vi "Draw Scale.vi"(6 "scale color":u32(colorbox), 9 "draw area cache":T1, 10 "heading (deg)":dbl, 11 "picture in":picture) -> (3 "picture out":picture)   [LabVIEW 2017, in "NI_Robotics_Compass Picture.lvlib"]
uses:
  <vilib>/robotics/Controls/Compass Indicator/Compass Picture/NI_Robotics_Compass Picture.lvlib
  <vilib>/robotics/Controls/Compass Indicator/Compass Picture/Draw Area State.ctl
  <vilib>/Utility/miscctls.llb/LVBoundsTypeDef.ctl
  <vilib>/picture/picture.llb/Draw Text at Point.vi
  <vilib>/picture/picture.llb/Draw Multiple Lines.vi
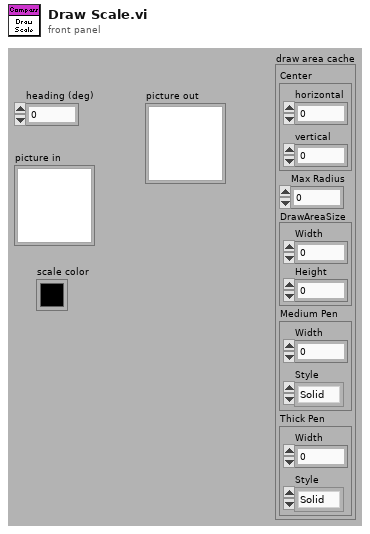
[diagram p1: front panel]
types:
  T1 = typedef "NI_Robotics_Compass Picture.lvlib/Draw Area State.ctl" = cluster{"Center":cluster{"horizontal":i16, "vertical":i16}, "Max Radius":dbl, "DrawAreaSize":T2, "Medium Pen":cluster{"Width":u16, "Style":enum32{"Solid", "Dash", "Dot", "DashDot", "DashDotDot"}}, "Thick Pen":cluster{"Width":u16, "Style":enum32{"Solid", "Dash", "Dot", "DashDot", "DashDotDot"}}}
  T2 = typedef "LVBoundsTypeDef.ctl" = cluster{"Width":u32, "Height":u32}
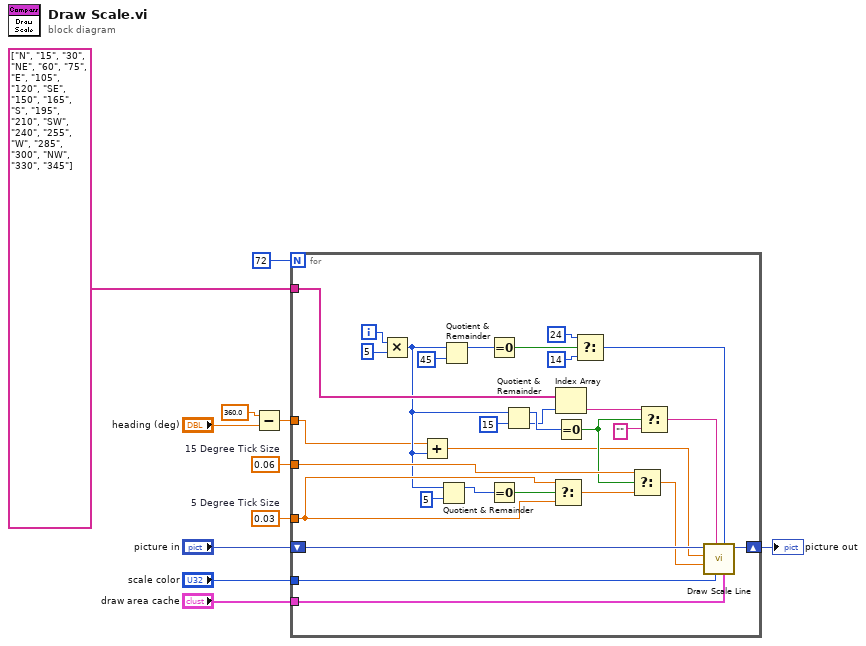
[diagram p0: block diagram]
diagram:
  w4 = 0.06  # 15 Degree Tick Size
  w3 = 0.03  # 5 Degree Tick Size
  n1 = Subtract(x=360.0, y="heading (deg)") -> (x-y=w10:dbl)
  n2 = for {
    N: 72 -> [_]
    tunnel: w3 -> [w23]
    tunnel: w4 -> [w35]
    shift-right: [w34] -> w5
    shift-left: "picture in" -> [w33]
    tunnel: string[] ["N", "15", "30", "NE", "60", "75", "E", "105", "120", "SE", "150", "165", "S", "195", "210", "SW", "240", "255", "W", "285", "300", "NW", "330", "345"] -> [w31]
    tunnel: w10 -> [w14]
    tunnel: "scale color" -> [w13]
    tunnel: "draw area cache" -> [w12]
    i -> [w25]
    n3 = Multiply(x=w25, y=5) -> (x*y=w16:i32)
    n4 = Add(x=w14, y=w16) -> (x+y=w15:dbl)
    n5 = Quotient & Remainder(x=w16, y=5) -> (x-y*floor(x/y)=w39:i32)  [unwired: 1 out]
    n6 = Quotient & Remainder(x=w16, y=45) -> (x-y*floor(x/y)=w22:i32)  [unwired: 1 out]
    n7 = Equal To 0?(x=w22) -> (x = 0?=w20:bool)
    n8 = Equal To 0?(x=w39) -> (x = 0?=w37:bool)
    n9 = Quotient & Remainder(x=w16, y=15) -> (x-y*floor(x/y)=w38:i32, floor(x/y)=w30:i32)
    n10 = Select(t=w23, s=w37, f=w23) -> (s? t:f=w36:dbl)
    n11 = Index Array(array=w31, index=w30) -> (element=w29:string)
    n12 = Equal To 0?(x=w38) -> (x = 0?=w28:bool)
    n13 = Select(t=24 ("y"), s=w20, f=14 ("y")) -> (s? t:f=w19:i32)
    n14 = Select(t=w35, s=w28, f=w36) -> (s? t:f=w32:dbl)
    n15 = Select(t=w29, s=w28, f="") -> (s? t:f=w26:string)
    n16 = call <vilib>:"Draw Scale Line.vi"("draw area cache"=w12, "font size"=w19, "scale color"=w13, "scale label"=w26, "line size (0-1)"=w32, "heading (rad)"=w15, "picture in"=w33) -> ("picture out"=w34:picture)  [unwired: 4 in]
  }
  "picture out" <- w5
